vi "CSM - Start Async Call.vi"   [LabVIEW 2014, in "Communicable State Machine.lvlib"]
doc: "VI snippet for dropping start async call template code from LabVIEW Quick Drop.\n\n<b>Inputs:</b>\n - N/A\n\n<b>Outputs:</b>\n - N/A"
uses:
  Communicable State Machine.lvlib
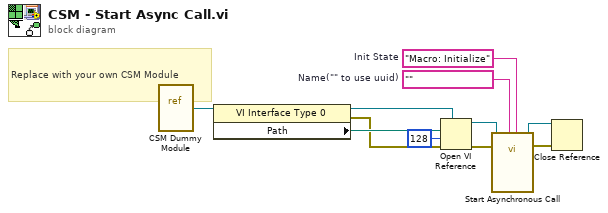
[diagram p0: block diagram]
diagram:
  w1 = "Macro: Initialize"  # Init State
  w5 = ""  # Name("" to use uuid)
  # "Replace with your own CSM Module"
  n1 = vi-ref "CSM Dummy Module.vi"() -> (w10:refnum<vi>)
  n2 = property class="VI Interface Type 0"(reference=w10) -> (reference out=w6:refnum<vi>, error out=w8:errorcluster, "Path"=w9:path)  [unwired: 1 in]
  n3 = Open VI Reference(type specifier VI Refnum (for type only)=w6, vi path=w9, options=128, error in (no error)=w8) -> (vi reference=w7:refnum<vi>, error out=w11:errorcluster)  [unwired: 2 in]
  n4 = call-by-ref "Start Asynchronous Call"(reference=w7, error in=w11, "Init State(\"Macro: Initialize\")"=w1, "Name(\"\" to use uuid)"=w5) -> (reference out=w3:refnum<vi>, error out=w4:errorcluster)  [unwired: 10 in]
  n5 = Close Reference(reference=w3, error in (no error)=w4) -> ()  [unwired: 1 out]
